vi "DIMPowerSupply.emergency off.vi"(0 "i ref in":refnum<vi>, 3 "ms timeout (10000)":i32=10000, 5 "error in (no error)":errorcluster) -> (14 "i ref out":refnum<vi>, 17 "timed out":bool, 19 "error out":errorcluster)   [LabVIEW 2014, in "DIMPowerSupply.lvlib"]
doc: "Performs an \"emergency off\" by setting the voltage to \"0\"."
uses:
  DIMPowerSupply.lvlib
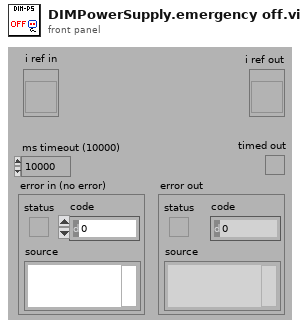
[diagram p1: front panel]
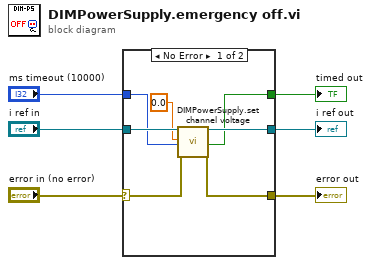
[diagram p0: block diagram]
diagram:
  n1 = case shown="No Error" "error in (no error)" {
    selector: "error in (no error)" -> [w9 w14]
    tunnel: [w8 w14] -> w6
    tunnel: [w12 w15] -> w5
    tunnel: "ms timeout (10000)" -> [w11 _]
    tunnel: "i ref in" -> [w13 w15]
    tunnel: [w10 _] -> w1
    frame No Error {
      n2 = call "DIMPowerSupply.set channel voltage.vi"("i ref in"=w13, "Voltage"=0.0, "ms timeout (10000)"=w11, "error in (no error)"=w9) -> ("i ref out"=w12:refnum<vi>, "timed out"=w10:bool, "error out"=w8:errorcluster)  [unwired: 13 in]
    }
    frame Error {
    }
  }
  "error out" <- w6
  "i ref out" <- w5
  "timed out" <- w1
